vi "Lab Ventilation.vi"(1 "Ventilation %":dbl) -> (0 "Scan Comments":string)   [LabVIEW 2017]
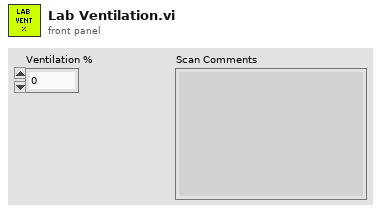
[diagram p1: front panel]
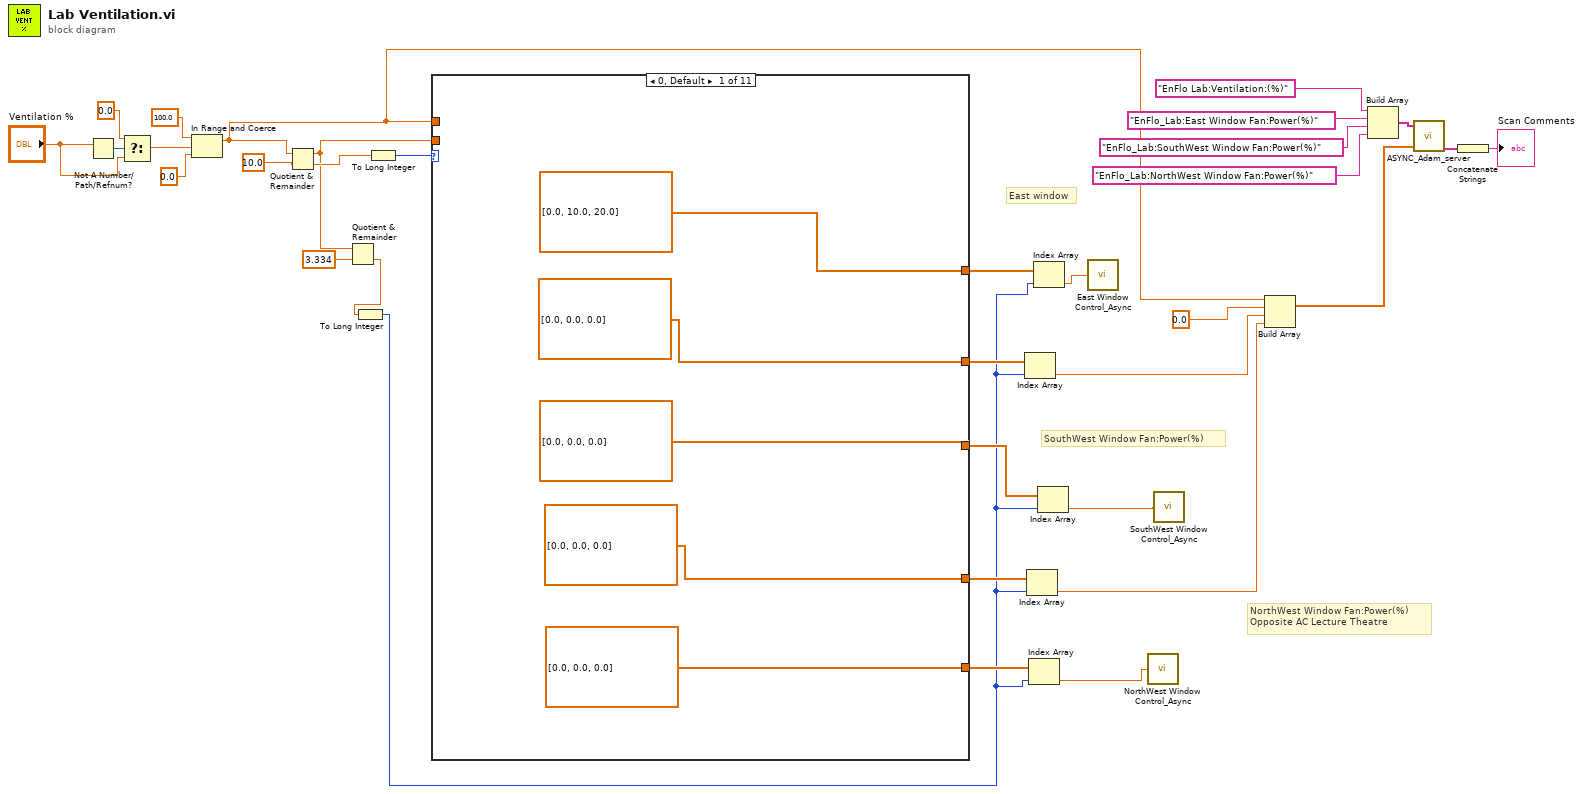
[diagram p0: block diagram]
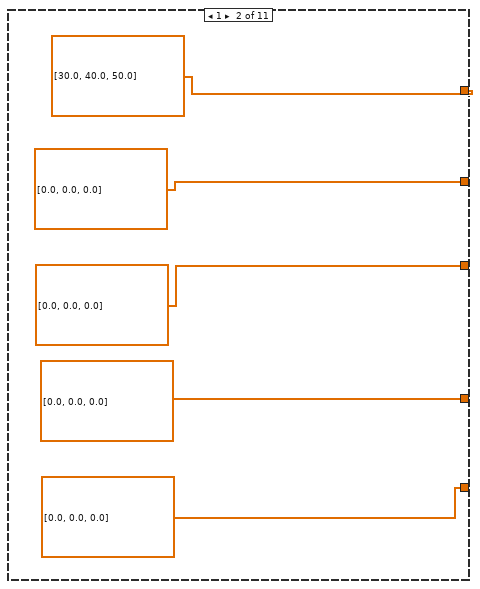
[diagram p2: hidden frame]
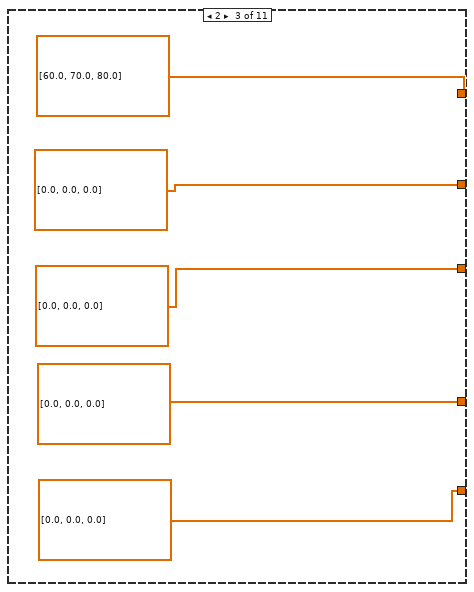
[diagram p3: hidden frame]
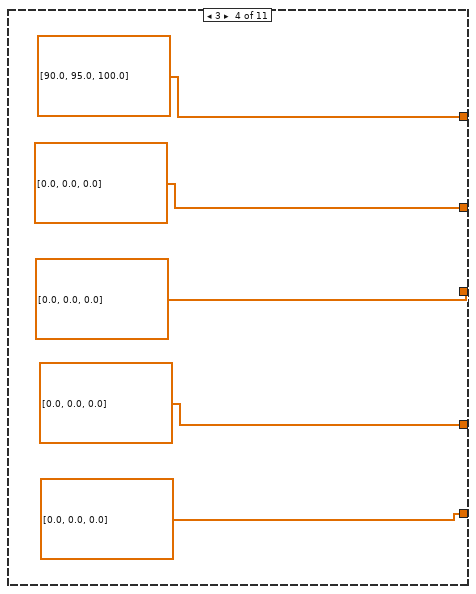
[diagram p4: hidden frame]
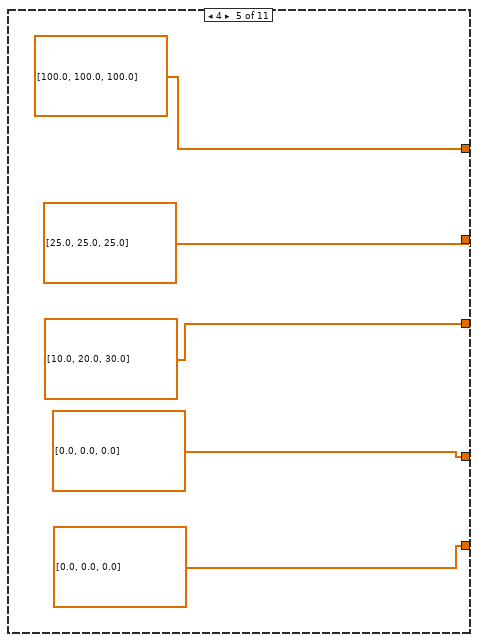
[diagram p5: hidden frame]
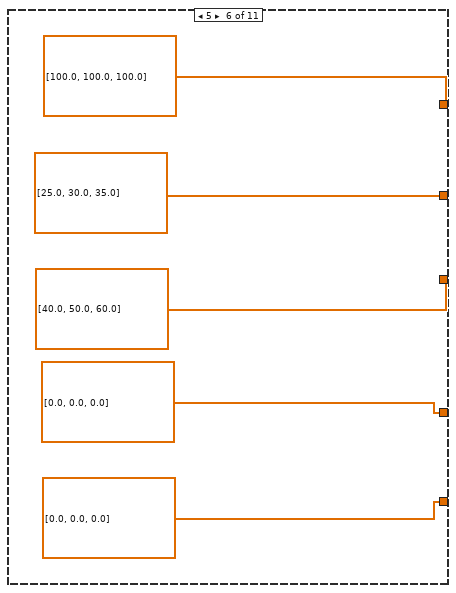
[diagram p6: hidden frame]
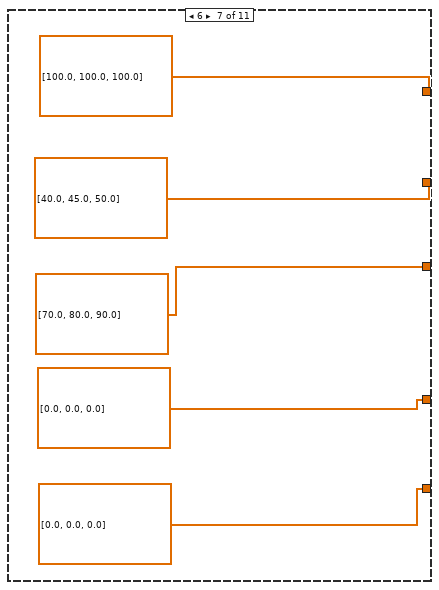
[diagram p7: hidden frame]
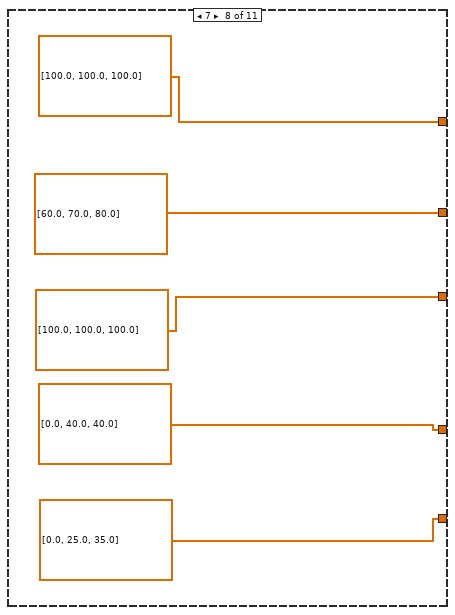
[diagram p8: hidden frame]
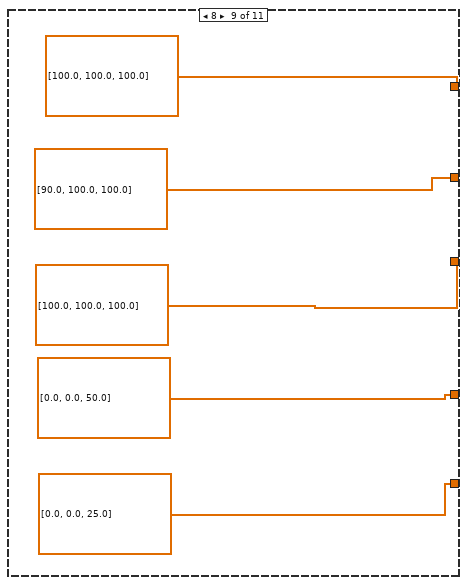
[diagram p9: hidden frame]
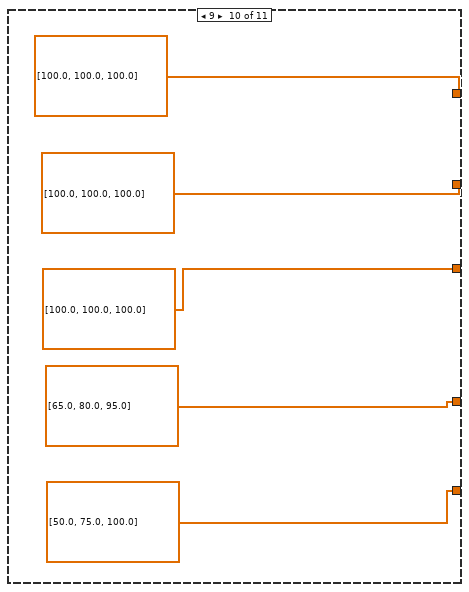
[diagram p10: hidden frame]
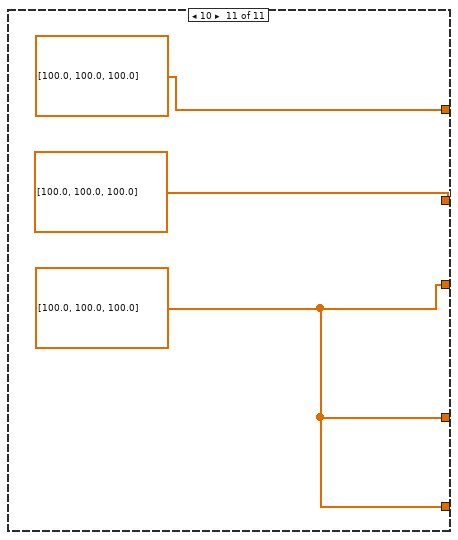
[diagram p11: hidden frame]
diagram:
  # "NorthWest Window Fan:Power(%)\nOpposite AC Lecture Theatre"
  # "SouthWest Window Fan:Power(%)"
  # "East window"
  n1 = Not A Number/Path/Refnum?(number/path/refnum="Ventilation %") -> (NaN/Path/Refnum?=w24:bool)
  n2 = Select(t=0.0, s=w24, f="Ventilation %") -> (s? t:f=w19:dbl)
  n3 = In Range and Coerce(upper limit=100.0, x=w19, lower limit=0.0) -> (coerced(x)=w18:dbl)  [unwired: 1 out]
  n4 = Quotient & Remainder(x=w18, y=10.0) -> (x-y*floor(x/y)=w17:dbl, floor(x/y)=w27:dbl)
  n5 = Quotient & Remainder(x=w17, y=3.334) -> (floor(x/y)=w15:dbl)  [unwired: 1 out]
  n6 = To Long Integer(number=w15) -> (32bit integer=w3:i32)
  n7 = To Long Integer(number=w27) -> (32bit integer=w33:i32)
  n8 = case shown="0, Default" w33 {
    tunnel: w18 -> [_ _ _ _ _ _ _ _ _ _ _]
    tunnel: w17 -> [_ _ _ _ _ _ _ _ _ _ _]
    tunnel: [dbl[] [0.0, 0.0, 0.0] ("appended array") dbl[] [0.0, 0.0, 0.0] ("appended array") dbl[] [0.0, 0.0, 0.0] ("appended array") dbl[] [0.0, 0.0, 0.0] ("appended array") dbl[] [25.0, 25.0, 25.0] ("appended array") dbl[] [25.0, 30.0, 35.0] ("appended array") dbl[] [40.0, 45.0, 50.0] ("appended array") dbl[] [60.0, 70.0, 80.0] ("appended array") dbl[] [90.0, 100.0, 100.0] ("appended array") dbl[] [100.0, 100.0, 100.0] ("appended array") dbl[] [100.0, 100.0, 100.0] ("appended array")] -> w14
    tunnel: [dbl[] [0.0, 0.0, 0.0] ("appended array") dbl[] [0.0, 0.0, 0.0] ("appended array") dbl[] [0.0, 0.0, 0.0] ("appended array") dbl[] [0.0, 0.0, 0.0] ("appended array") dbl[] [10.0, 20.0, 30.0] ("appended array") dbl[] [40.0, 50.0, 60.0] ("appended array") dbl[] [70.0, 80.0, 90.0] ("appended array") dbl[] [100.0, 100.0, 100.0] ("appended array") dbl[] [100.0, 100.0, 100.0] ("appended array") dbl[] [100.0, 100.0, 100.0] ("appended array") w84] -> w13
    tunnel: [dbl[] [0.0, 10.0, 20.0] ("appended array") dbl[] [30.0, 40.0, 50.0] ("appended array") dbl[] [60.0, 70.0, 80.0] ("appended array") dbl[] [90.0, 95.0, 100.0] ("appended array") dbl[] [100.0, 100.0, 100.0] ("appended array") dbl[] [100.0, 100.0, 100.0] ("appended array") dbl[] [100.0, 100.0, 100.0] ("appended array") dbl[] [100.0, 100.0, 100.0] ("appended array") dbl[] [100.0, 100.0, 100.0] ("appended array") dbl[] [100.0, 100.0, 100.0] ("appended array") dbl[] [100.0, 100.0, 100.0] ("appended array")] -> w11
    tunnel: [dbl[] [0.0, 0.0, 0.0] ("appended array") dbl[] [0.0, 0.0, 0.0] ("appended array") dbl[] [0.0, 0.0, 0.0] ("appended array") dbl[] [0.0, 0.0, 0.0] ("appended array") dbl[] [0.0, 0.0, 0.0] ("appended array") dbl[] [0.0, 0.0, 0.0] ("appended array") dbl[] [0.0, 0.0, 0.0] ("appended array") dbl[] [0.0, 40.0, 40.0] ("appended array") dbl[] [0.0, 0.0, 50.0] ("appended array") dbl[] [65.0, 80.0, 95.0] ("appended array") w84] -> w5
    tunnel: [dbl[] [0.0, 0.0, 0.0] ("appended array") dbl[] [0.0, 0.0, 0.0] ("appended array") dbl[] [0.0, 0.0, 0.0] ("appended array") dbl[] [0.0, 0.0, 0.0] ("appended array") dbl[] [0.0, 0.0, 0.0] ("appended array") dbl[] [0.0, 0.0, 0.0] ("appended array") dbl[] [0.0, 0.0, 0.0] ("appended array") dbl[] [0.0, 25.0, 35.0] ("appended array") dbl[] [0.0, 0.0, 25.0] ("appended array") dbl[] [50.0, 75.0, 100.0] ("appended array") w84] -> w4
    frame 0, Default {
    }
    frame 1 {
    }
    frame 2 {
    }
    frame 3 {
    }
    frame 4 {
    }
    frame 5 {
    }
    frame 6 {
    }
    frame 7 {
    }
    frame 8 {
    }
    frame 9 {
    }
    frame 10 {
      w84 = dbl[] [100.0, 100.0, 100.0] ("appended array")
    }
  }
  n9 = Index Array(array=w14, index=w3) -> (element=w6:dbl)
  n10 = Index Array(array=w5, index=w3) -> (element=w2:dbl)
  n11 = Index Array(array=w4, index=w3) -> (element=w1:dbl)
  n12 = Index Array(array=w11, index=w3) -> (element=w12:dbl)
  n13 = Index Array(array=w13, index=w3) -> (element=w10:dbl)
  n14 = call "East Window Control_Async.vi"("Desired Window Open %"=w12) -> ()  [unwired: 1 in]
  n15 = call "NorthWest Window Control_Async.vi"("Desired Window Open %"=w1) -> ()  [unwired: 1 in]
  n16 = call "SouthWest Window Control_Async.vi"("Desired Window Open %"=w10) -> ()  [unwired: 1 in]
  n17 = Build Array(w18, 0.0 ("element"), w6, w2) -> (w29:dbl[])
  n18 = Build Array("EnFlo Lab:Ventilation:(%)", "EnFlo_Lab:East Window Fan:Power(%)", "EnFlo_Lab:SouthWest Window Fan:Power(%)", "EnFlo_Lab:NorthWest Window Fan:Power(%)") -> (w30:string[])
  n19 = call "ASYNC_Adam_server.vi"("Values"=w29, "Channel Names"=w30) -> ("Scan Comments"=w26:string[])  [unwired: 1 in, 2 out]
  n20 = Concatenate Strings(w26) -> (→"Scan Comments":string)
